vi "1dg UI.vi"(10 "String":string) -> ()   [LabVIEW 2024, in "FormulaG.lvlib" / "FormulaG App.lvclass"]
uses:
  FormulaG App.lvclass
panel:
  in  "Boolean":bool
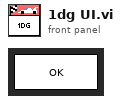
[diagram p1: front panel]
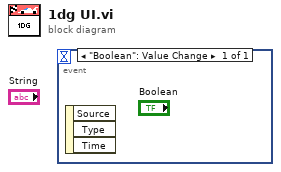
[diagram p0: block diagram]
diagram:
  n1 = event shown="[0] \"Boolean\": Value Change" {
    selector: _ -> [_]
    dyn-events: _ -> [_]
    timeout: _ -> [_]
    event "Boolean": Value Change {
      n2 = event-data() -> ()  [unwired: 1 in, 3 out]
    }
  }
